vi "Main Menu.vi"() -> ()   [LabVIEW 2017]
uses:
  Controls/Main Menu States.ctl
panel:
  out "Frequency 2":dbl
  out "Frequency":dbl
  in  "Stop Button":bool
  in  "Name Button":bool
  in  "Calibrate Button":bool
  out "Mic 2":dynamicdata(graph)
  out "Sensor 6":dynamicdata(graph)
  out "Sensor 4":dynamicdata(graph)
  out "Sensor 2":dynamicdata(graph)
  out "Mic 1":dynamicdata(graph)
  out "Sensor 5":dynamicdata(graph)
  out "Sensor 3":dynamicdata(graph)
  out "Sensor 1":dynamicdata(graph)
  in  "Analysis Button":bool
  in  "Record Button":bool
  out "Message to User":string
  in  "Exit Button":bool
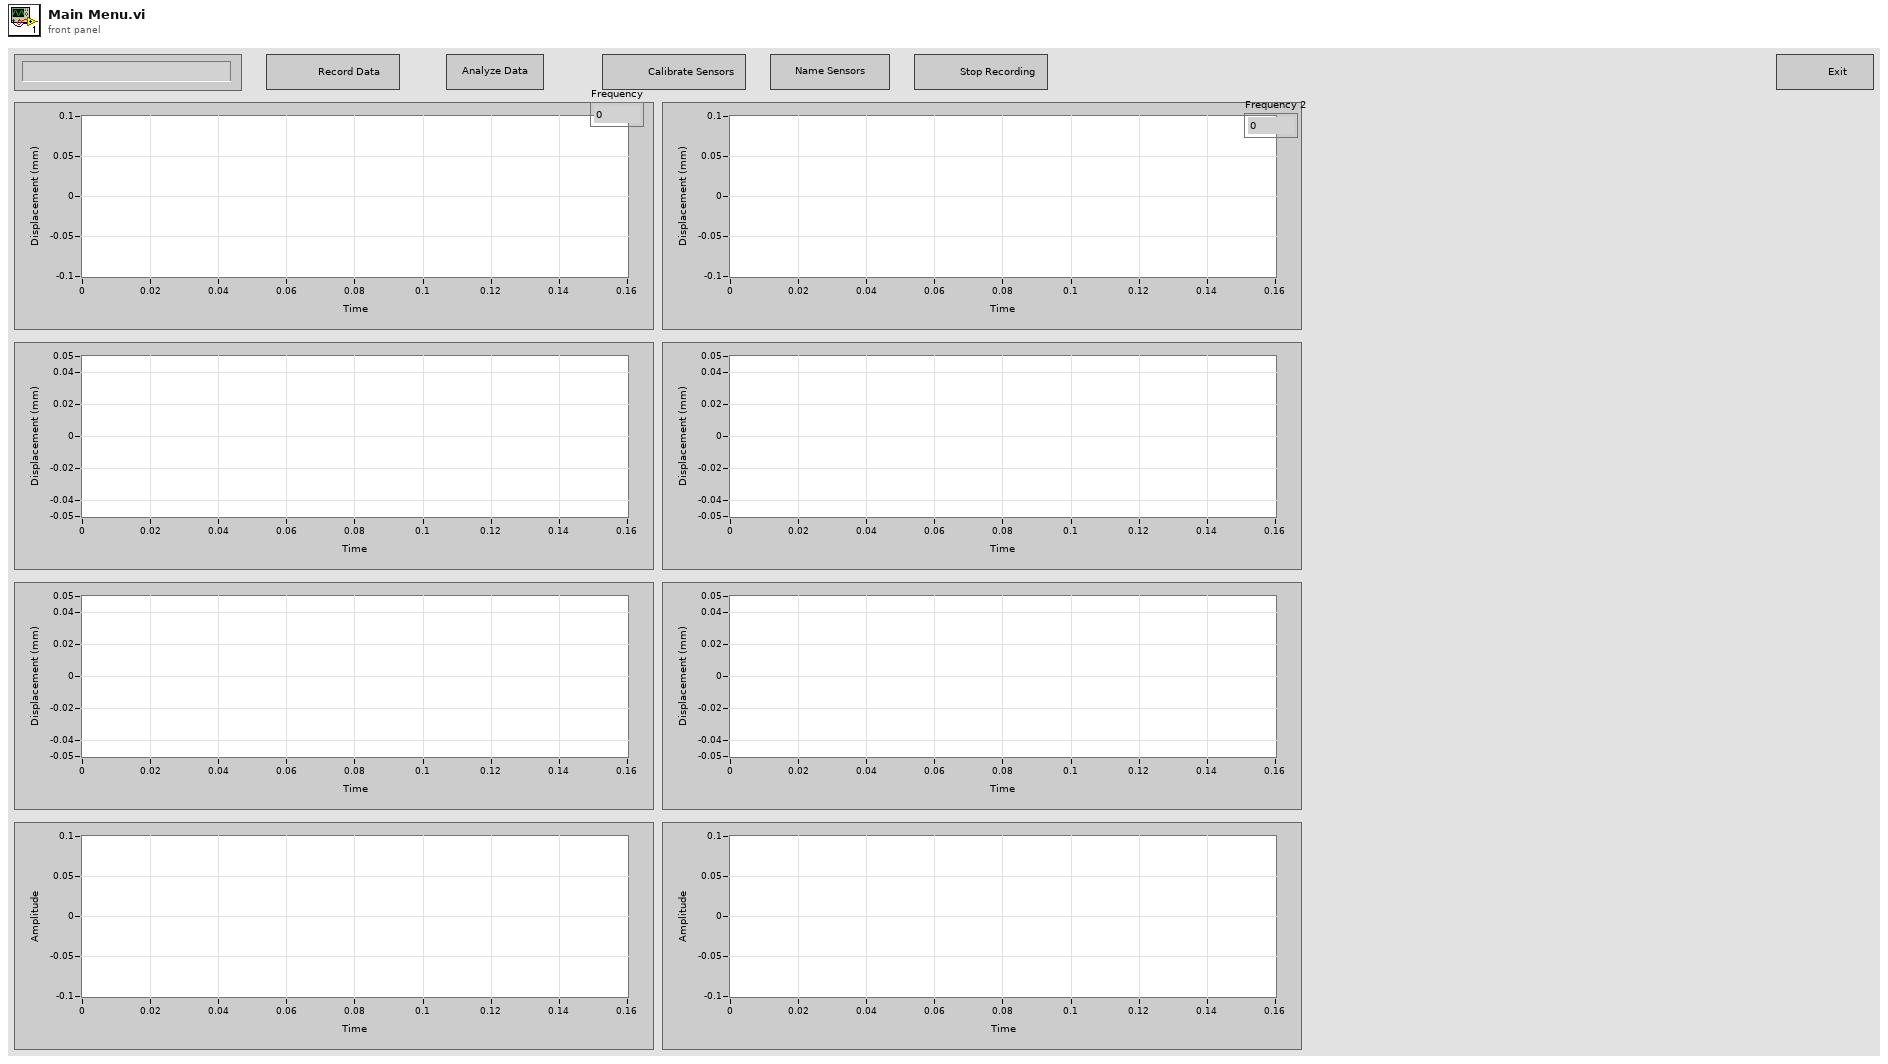
[diagram p1: front panel]
types:
  T1 = typedef "Main Menu States.ctl" = enum16{"Initialize", "Update UI", "Wait", "Collect", "Analyze", "Exit"}
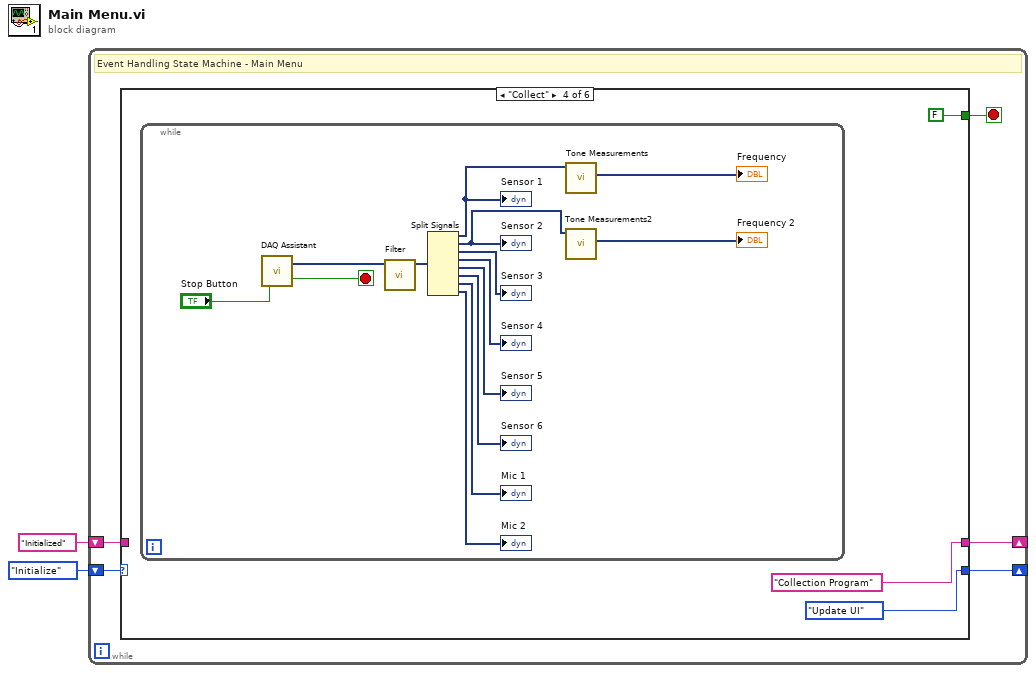
[diagram p0: block diagram]
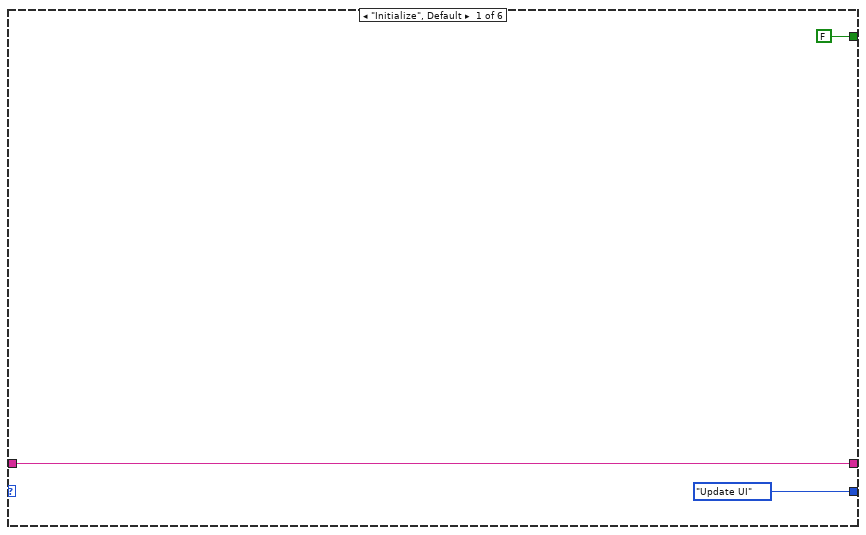
[diagram p2: hidden frame]
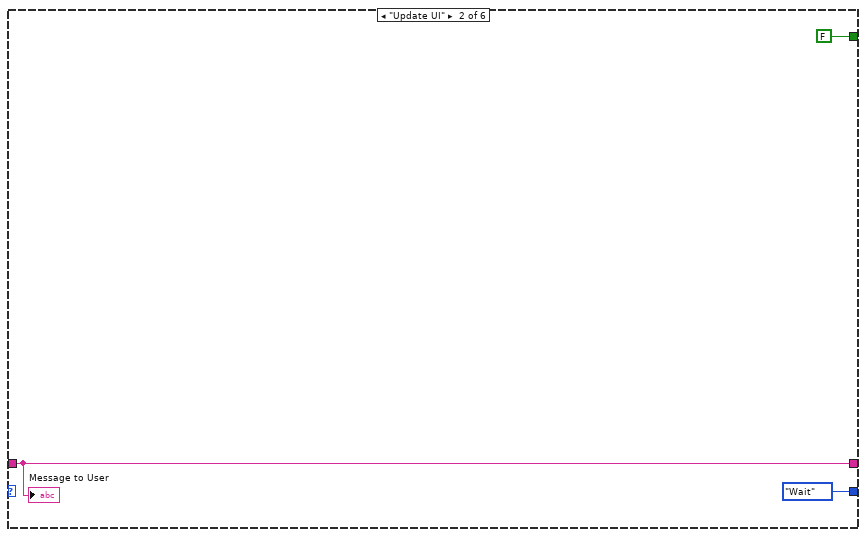
[diagram p3: hidden frame]
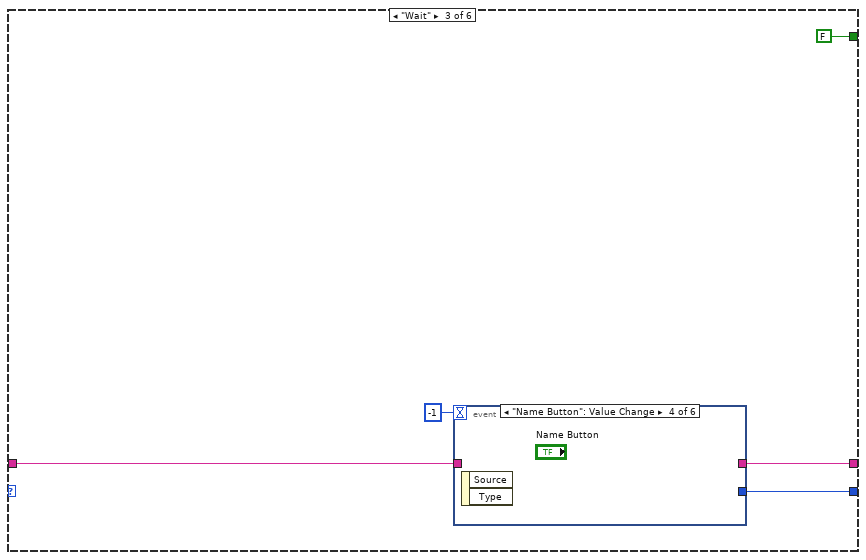
[diagram p4: hidden frame]
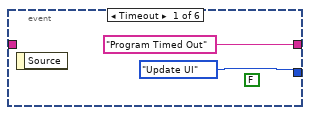
[diagram p5: hidden frame]
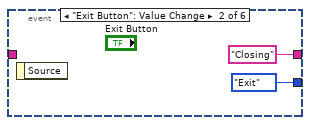
[diagram p6: hidden frame]
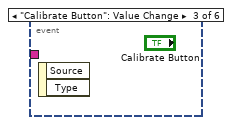
[diagram p7: hidden frame]
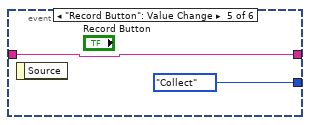
[diagram p8: hidden frame]
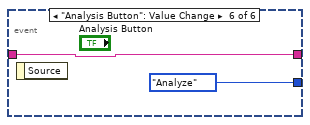
[diagram p9: hidden frame]
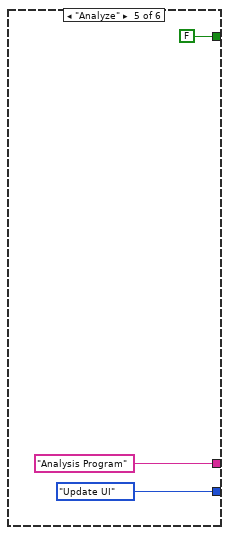
[diagram p10: hidden frame]
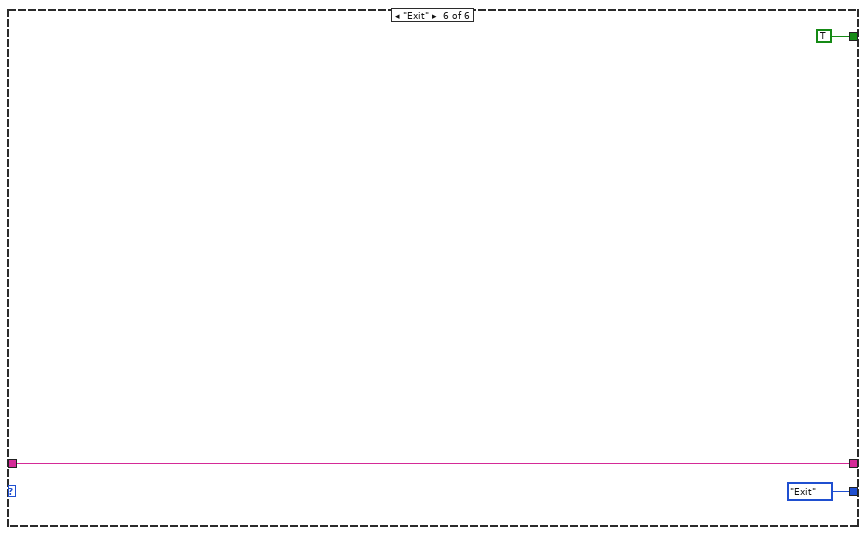
[diagram p11: hidden frame]
diagram:
  n1 = while {
    shift-right: [w5] -> _
    shift-left: Main_Menu_States."Initialize" -> [w6]
    shift-right: [w3] -> _
    shift-left: "Initialized" ("Message to User") -> [w4]
    stop <- w7 stop-if-true
    # "Event Handling State Machine - Main Menu"
    n2 = case shown="\"Collect\"" w6 {
      tunnel: [FALSE FALSE FALSE FALSE FALSE TRUE] -> w7
      tunnel: [Main_Menu_States."Update UI" Main_Menu_States."Wait" w17 Main_Menu_States."Update UI" Main_Menu_States."Update UI" Main_Menu_States."Exit"] -> w5
      tunnel: w4 -> [w8 w12 w15 _ _ w47]
      tunnel: [w8 w12 w16 "Collection Program" ("Message to User") "Analysis Program" ("Message to User 2") w47] -> w3
      frame "Initialize", Default {
      }
      frame "Update UI" {
        "Message to User" <- w12
      }
      frame "Wait" {
        n3 = event shown="[3] \"Name Button\": Value Change" {
          selector: _ -> [_ _ _ _ _ _]
          dyn-events: _ -> [_ _ _ _ _ _]
          timeout: -1 -> [_ _ _ _ _ _]
          tunnel: [Main_Menu_States."Update UI" Main_Menu_States."Exit" _ _ Main_Menu_States."Collect" Main_Menu_States."Analyze"] -> w17
          tunnel: ["Program Timed Out" ("Message to User") "Closing" ("Message to User") _ _ w24 w25] -> w16
          tunnel: w15 -> [_ _ _ _ w24 w25]
          event Timeout {
            (unwired) FALSE
            n4 = event-data() -> ()  [unwired: 1 in, 1 out]
          }
          event "Exit Button": Value Change {
            n5 = event-data() -> ()  [unwired: 1 in, 1 out]
          }
          event "Calibrate Button": Value Change {
            n6 = event-data() -> ()  [unwired: 1 in, 2 out]
          }
          event "Name Button": Value Change {
            n7 = event-data() -> ()  [unwired: 1 in, 2 out]
          }
          event "Record Button": Value Change {
            n8 = event-data() -> ()  [unwired: 1 in, 1 out]
          }
          event "Analysis Button": Value Change {
            n9 = event-data() -> ()  [unwired: 1 in, 1 out]
          }
        }
      }
      frame "Collect" {
        n10 = while {
          stop <- w42 stop-if-true
          n11 = call "DAQ Assistant"("stop (F)"="Stop Button") -> ("data"=w35:dynamicdata, "stopped"=w42:bool)  [unwired: 15 in, 2 out]
          n12 = call "Filter"("Signal"=w35) -> ("Filtered Signal"=w34:dynamicdata)  [unwired: 9 in, 1 out]
          n13 = Split Signals(w34) -> (w33:dynamicdata, w31:dynamicdata, →"Sensor 3":dynamicdata, →"Sensor 4":dynamicdata, →"Sensor 5":dynamicdata, →"Sensor 6":dynamicdata, →"Mic 1":dynamicdata, →"Mic 2":dynamicdata)  [unwired: 8 in]
          "Sensor 1" <- w33
          "Sensor 2" <- w31
          n14 = call "Tone Measurements"("Signals"=w33) -> ("Frequency"=→"Frequency":dynamicdata)  [unwired: 8 in, 2 out]
          n15 = call "Tone Measurements2"("Signals"=w31) -> ("Frequency"=→"Frequency 2":dynamicdata)  [unwired: 8 in, 2 out]
        }
      }
      frame "Analyze" {
      }
      frame "Exit" {
      }
    }
  }
